vi "get play mode ring.vi"(8 "error in (no error)":errorcluster caption="에러 입력(에러 없음)", 11 "DW7802 입력":refnum<class "DW7802.lvclass">) -> (0 "error out":errorcluster caption="에러 출력", 1 "caption":string="Play Mode", 2 "strings & values":T1=[{"String"="Direct Playback Mode", "Value"=0}, {"String"="Synthesis Playback Mode", "Value"=1}], 3 "DW7802 출력":refnum<class "DW7802.lvclass">, 4 "default value":u8, 6 "using":bool=TRUE)   [LabVIEW 2020, in "DW7802.lvclass"]
uses:
  DW7802.lvclass
  <vilib>/Utility/miscctls.llb/LVStringsAndValuesArrayTypeDef_U8.ctl
  Haptic IC/Haptic IC.lvclass
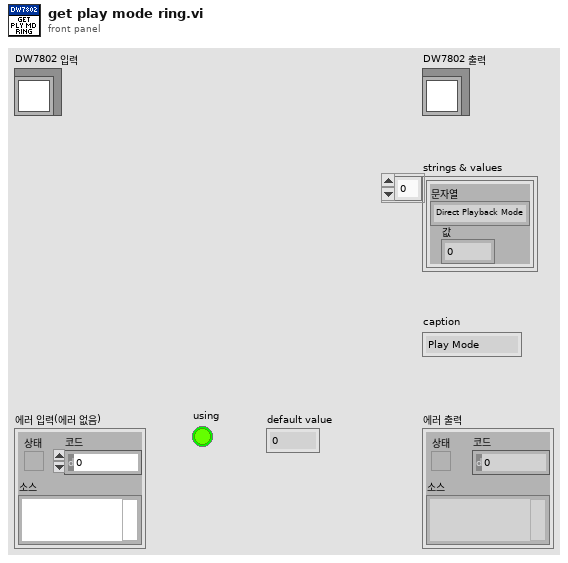
[diagram p1: front panel]
types:
  T1 = typedef "LVStringsAndValuesArrayTypeDef_U8.ctl" = cluster{"String":string, "Value":u8}[]
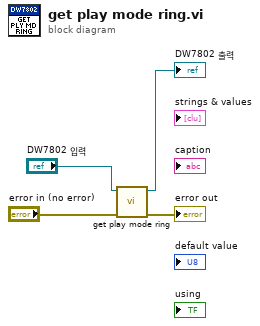
[diagram p0: block diagram]
diagram:
  n1 = call-parent "get play mode ring.vi"("error in (no error)"="error in (no error)", "Haptic IC 입력"="DW7802 입력") -> ("error out"=→"error out":errorcluster, "Haptic IC 출력"=→"DW7802 출력":refnum<class "DW7802.lvclass">)  [unwired: 4 in, 4 out]
